vi "change tag type.vi"(7 "owner ID":string, 8 "error in":errorcluster, 9 "new data type":T1, 10 "tag name":string, 11 "engine configuration in":refnum<class "engine configuration.lvclass">) -> (0 "error out":errorcluster, 3 "engine configuration out":refnum<class "engine configuration.lvclass">)   [LabVIEW 2013, in "engine configuration.lvclass"]
uses:
  engine configuration.lvclass
  <vilib>/NI/Tag Bus/tag/Data Type.ctl
  <vilib>/NI/Tag Bus/tag/tag descriptor.lvclass
  <vilib>/NI/Tag Bus/tag/tag descriptor.lvclass/tag descriptor.ctl
  engine configuration.lvclass/engine configuration.ctl
  <vilib>/NI/Tag Bus/tag/write data type.vi
  <vilib>/NI/Tag Bus/tag/write tag name.vi
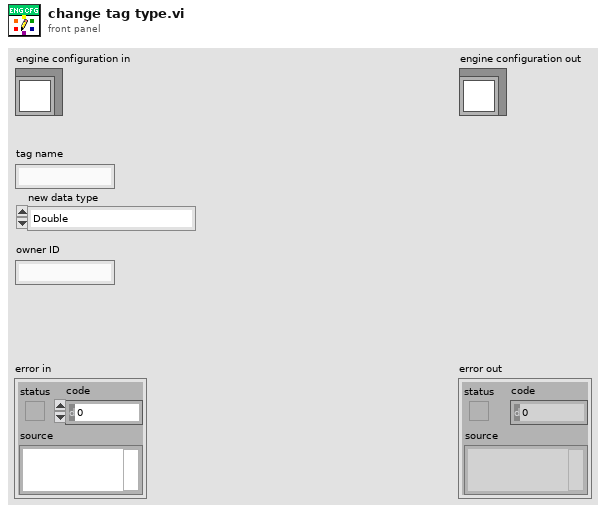
[diagram p1: front panel]
types:
  T1 = typedef "tag bus.lvlib/tag descriptor.lvclass/Data Type.ctl" = enum16{"Double", "Single", "I64", "I32", "I16", "I8", "U64", "U32", "U16", "U8", "Boolean", "String", "Array of Double", "Array of Single", "Array of I64", "Array of I32", "Array of I16", "Array of I8", "Array of U64", "Array of U32", "Array of U16", "Array of U8", "Array of Boolean", "Array of String"}
  T2 = typedef "engine configuration.lvclass/Tag Info.ctl" = cluster{"Tag":refnum<class "tag descriptor.lvclass">, "Writer":string, "Readers":string[], "Owning ID":string}
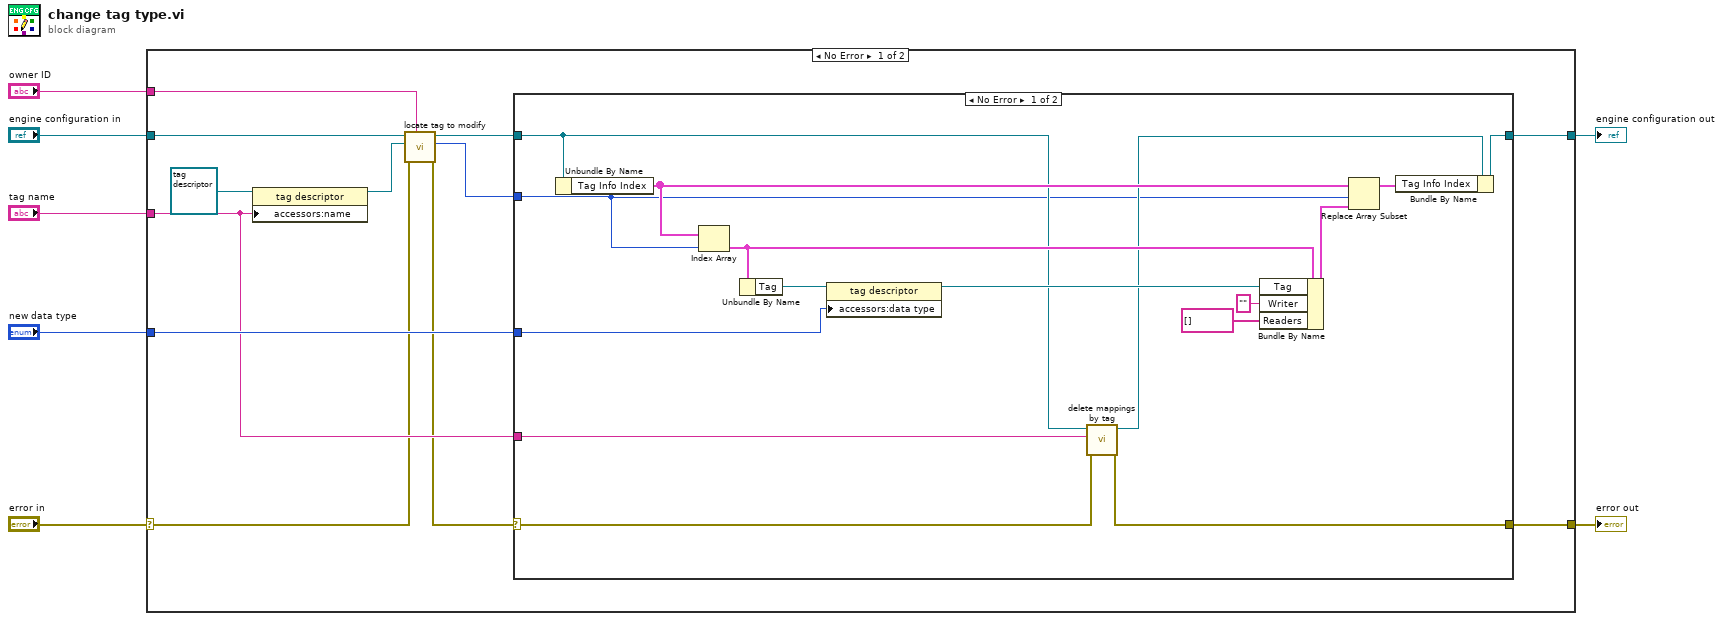
[diagram p0: block diagram]
diagram:
  n1 = case shown="No Error" "error in" {
    selector: "error in" -> [w10 w39]
    tunnel: [w17 w39] -> w6
    tunnel: [w18 w38] -> w4
    tunnel: "engine configuration in" -> [w14 w38]
    tunnel: "tag name" -> [w15 _]
    tunnel: "new data type" -> [w16 _]
    tunnel: "owner ID" -> [w11 _]
    frame No Error {
      n2 = property class="tag descriptor"(reference=refnum<class "tag descriptor.lvclass"> refnum ("tag descriptor"), "accessors:name"=w15) -> (reference out=w12:refnum<class "tag descriptor.lvclass">)  [unwired: 1 in, 1 out]
      n3 = call "locate tag to modify.vi"("owner ID"=w11, "error in"=w10, "tag descriptor"=w12, "engine configuration in"=w14) -> ("error out"=w9:errorcluster, "index"=w8:i32, "engine configuration out"=w13:refnum<class "engine configuration.lvclass">)  [unwired: 5 in]
      n4 = case shown="No Error" w9 {
        selector: w9 -> [w20 w36]
        tunnel: w13 -> [w27 w37]
        tunnel: [w28 w37] -> w18
        tunnel: [w26 w36] -> w17
        tunnel: w16 -> [w34 _]
        tunnel: w15 -> [w24 _]
        tunnel: w8 -> [w21 _]
        frame No Error {
          n5 = Unbundle By Name(w27) -> ("Tag Info Index"=w31:T2[])
          n6 = Index Array(array=w31, index=w21) -> (element=w33:T2)
          n7 = Unbundle By Name(w33) -> ("Tag"=w35:refnum<class "tag descriptor.lvclass">)
          n8 = property class="tag descriptor"(reference=w35, "accessors:data type"=w34) -> (reference out=w32:refnum<class "tag descriptor.lvclass">)  [unwired: 1 in, 1 out]
          n9 = call "delete mappings by tag.vi"("error in"=w20, "tag name"=w24, "engine configuration in"=w27) -> ("error out"=w26:errorcluster, "engine configuration out"=w25:refnum<class "engine configuration.lvclass">)  [unwired: 7 in]
          n10 = Bundle By Name(cluster=w33, "Tag"=w32, "Writer"="", "Readers"=string[] []) -> (w30:T2)
          n11 = Replace Array Subset(array=w31, new element=w30, index=w21) -> (w29:T2[])
          n12 = Bundle By Name(cluster=w25, "Tag Info Index"=w29) -> (w28:refnum<class "engine configuration.lvclass">)
        }
        frame Error {
        }
      }
    }
    frame Error {
    }
  }
  "error out" <- w6
  "engine configuration out" <- w4
